vi "send tables number.vi"() -> ()   [LabVIEW 2018]
uses:
  <vilib>/Tufts CEEO ROS for LabVIEW Software/ROS/Code/SubVIs/_ROSControl.ctl
  <vilib>/Tufts CEEO ROS for LabVIEW Software/ROS/Code/SubVIs/_ROSDirection.ctl
  <vilib>/Tufts CEEO ROS for LabVIEW Software/ROS/Code/Console/Servers/ServerSubs/TopicDef.ctl
  <vilib>/Tufts CEEO ROS for LabVIEW Software/ROS/MessageBuilding/std_msgs/subs/stringScalar.vi
panel:
  out "ROS out":T1={"topic port"=0, "Node"="", "topic"="", "type"="", "node port"=0, "error "={"status"=FALSE, "code"=0, "source"=""}, "Direction"=enum."Node", "Update (ms)"=1, "FIFO size"=1}
  out "error out":errorcluster
  in  "stop":bool=TRUE
  in  "Send":bool
  in  "table 5":bool
  in  "table 4":bool
  in  "table 3":bool
  in  "table2":bool
  in  "table 1":bool
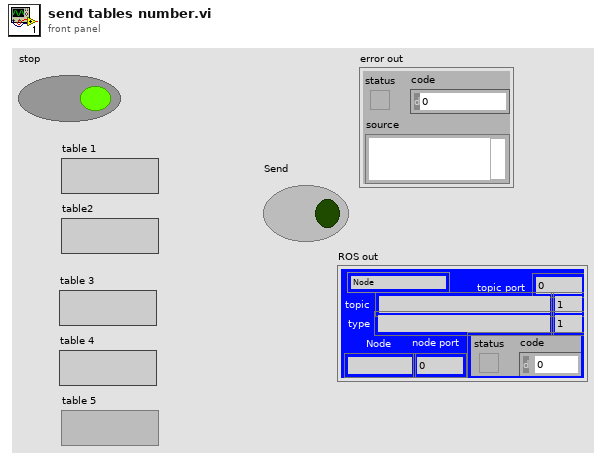
[diagram p1: front panel]
types:
  T1 = typedef "_ROSControl.ctl" = cluster{"topic port":u16, "Node":string, "topic":string, "type":string, "node port":u16, "error ":errorcluster, "Direction":T2, "Update (ms)":u16, "FIFO size":u16}
  T2 = typedef "_ROSDirection.ctl" = enum16{"Node", "Publisher", "Subscriber", "ServiceClient", "ServiceProvider"}
  T3 = typedef "TopicDef.ctl" = cluster{"Topic":string, "Type":string, "Action":T2, "Update (ms)":u16, "queue size":u16}
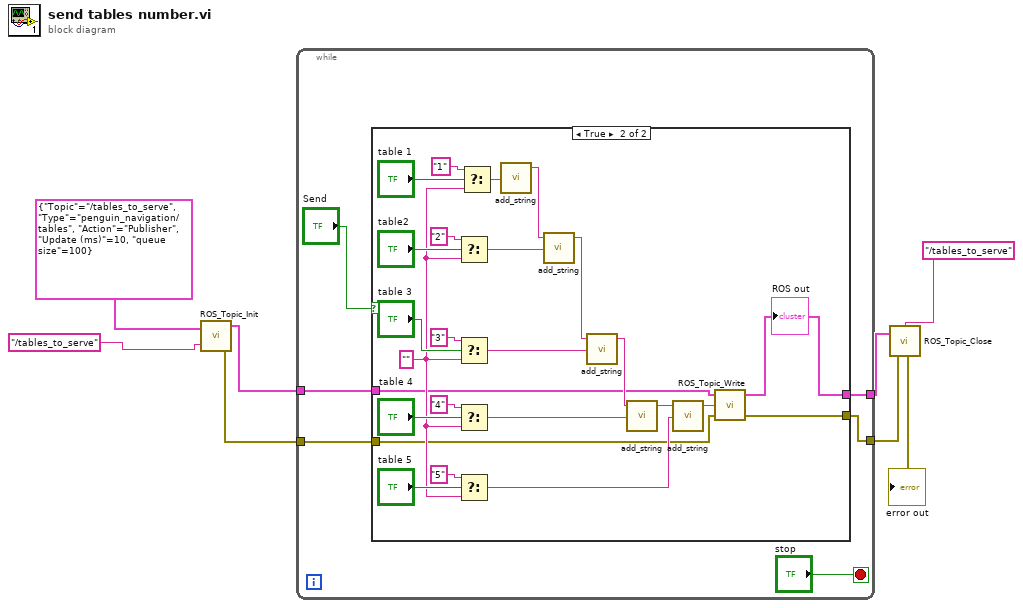
[diagram p0: block diagram]
diagram:
  n1 = call <vilib>:"ROS_Topic_Init.vi"("Definitions"=T3 {"Topic"="/tables_to_serve", "Type"="penguin_navigation/tables", "Action"=enum."Publisher", "Update (ms)"=10, "queue size"=100}, "node"="/tables_to_serve") -> ("ROS out"=w4:T1, "error out"=w3:errorcluster)  [unwired: 1 in]
  n2 = while {
    tunnel: [w13] -> w6
    tunnel: [w12] -> w7
    tunnel: w4 -> [w10]
    tunnel: w3 -> [w9]
    stop <- "stop" stop-if-true
    n3 = case shown="True" "Send" {
      tunnel: [w15 w22] -> w13
      tunnel: [w16 w21] -> w12
      tunnel: w10 -> [w16 w20]
      tunnel: w9 -> [w15 w19]
      frame False {
      }
      frame True {
        w32 = "" ("t")
        n4 = Select(t="2", s="table2", f=w32) -> (s? t:f=w27:string)
        n5 = Select(t="3", s="table 3", f=w32) -> (s? t:f=w26:string)
        n6 = Select(t="4", s="table 4", f=w32) -> (s? t:f=w25:string)
        n7 = Select(t="5", s="table 5", f=w32) -> (s? t:f=w24:string)
        n8 = Select(t="1", s="table 1", f=w32) -> (s? t:f=w30:string)
        n9 = call-poly <vilib>:"add_string.vi"("String"=w30) -> ("msg out"=w29:string)  [unwired: 4 in]
        n10 = call-poly <vilib>:"add_string.vi"("String"=w27, "msg in"=w29) -> ("msg out"=w28:string)  [unwired: 3 in]
        n11 = call-poly <vilib>:"add_string.vi"("String"=w26, "msg in"=w28) -> ("msg out"=w31:string)  [unwired: 3 in]
        n12 = call-poly <vilib>:"add_string.vi"("String"=w25, "msg in"=w31) -> ("msg out"=w17:string)  [unwired: 3 in]
        n13 = call-poly <vilib>:"add_string.vi"("String"=w24, "msg in"=w17) -> ("msg out"=w23:string)  [unwired: 3 in]
        n14 = call <vilib>:"ROS_Topic_Write.vi"("error in (no error)"=w19, "Msg in"=w23, "ROS in"=w20) -> ("error out"=w22:errorcluster, "ROS out"=w21:T1)  [unwired: 1 in]
        "ROS out" <- w21
      }
    }
  }
  n15 = call <vilib>:"ROS_Topic_Close.vi"("error in"=w6, "ROS in"=w7, "node"="/tables_to_serve") -> ("error out"=→"error out":errorcluster)  [unwired: 1 in]
